vi "3dLoad.vi"(11 "name or relative path":string="Hexa1.stl") -> (0 "Object":refnum<vi>, 1 "reference out":refnum<vi>, 3 "appended path 2":path)   [LabVIEW 2011]
uses:
  <vilib>/picture/3D Picture Control/NI_3D Picture Control.lvlib
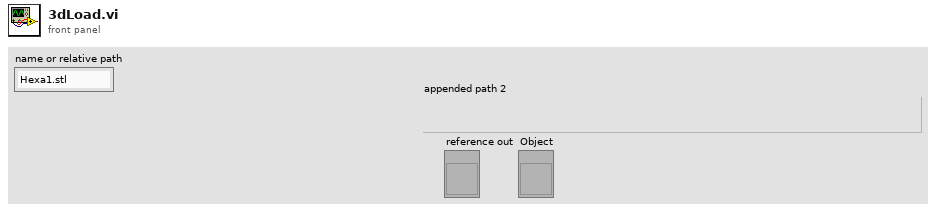
[diagram p1: front panel]
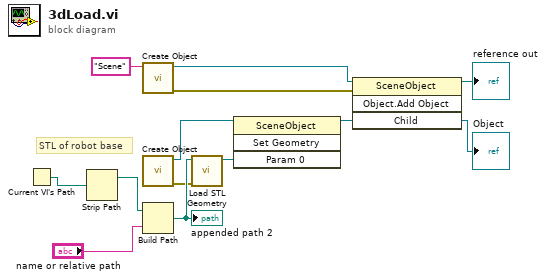
[diagram p0: block diagram]
diagram:
  # "STL of robot base"
  n1 = Current VI's Path() -> (path=w2:path)
  n2 = Strip Path(path=w2) -> (stripped path=w1:path)  [unwired: 1 out]
  n3 = call <vilib>:"Create Object.vi"("Name"="Scene") -> ("error out"=w13:errorcluster, "Scene:New Object"=w12:refnum<vi>)  [unwired: 9 in]
  n4 = call <vilib>:"Create Object.vi"() -> ("error out"=w7:errorcluster, "Scene:New Object"=w8:refnum<vi>)  [unwired: 10 in]
  n5 = Build Path(base path=w1, name or relative path="name or relative path") -> (appended path=w10:path)
  "appended path 2" <- w10
  n6 = call <vilib>:"Load STL Geometry.vi"("error in (no error)"=w7, "Model File"=w10) -> ("New Mesh Refnum"=w9:refnum<vi>)  [unwired: 8 in, 1 out]
  n7 = invoke class="SceneObject" method="Set Geometry"(reference=w8, "Param 0"=w9) -> (reference out=w6:refnum<vi>)  [unwired: 2 in, 3 out]
  n8 = invoke class="SceneObject" method="Object.Add Object"(reference=w12, error in=w13, "Child"=w6) -> (reference out=→"reference out":refnum<vi>, "Child"=→"Object":refnum<vi>)  [unwired: 1 in, 2 out]
